vi "Group_WriteLog.vi"(0 "Group in":refnum<class "Group.lvclass">, 1 "tdms file":refnum<k34>, 7 "Loop Counter":i32, 9 "t0":timestamp, 11 "error in (no error)":errorcluster, 12 "dt per loop":dbl) -> (4 "Group out":refnum<class "Group.lvclass">, 6 "tdms file out":refnum<k34>, 15 "error out":errorcluster)   [LabVIEW 2023, in "Group.lvclass"]
doc: "A mid level VI which trickles down to call the write method on all channels within this group."
uses:
  Group.lvclass
  Group.lvclass/Group.ctl
  Channel/Channel.lvclass
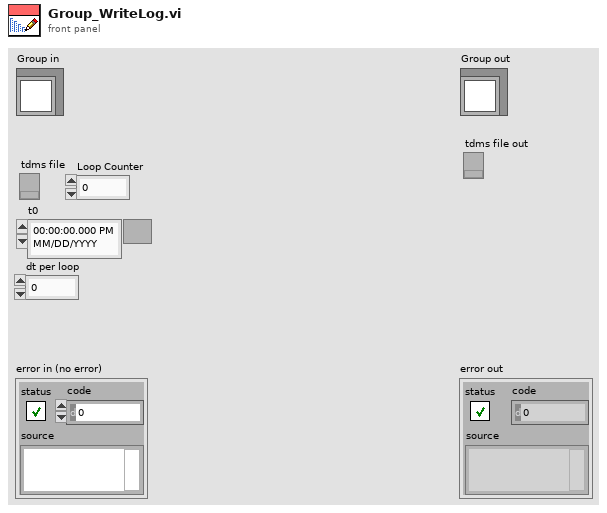
[diagram p1: front panel]
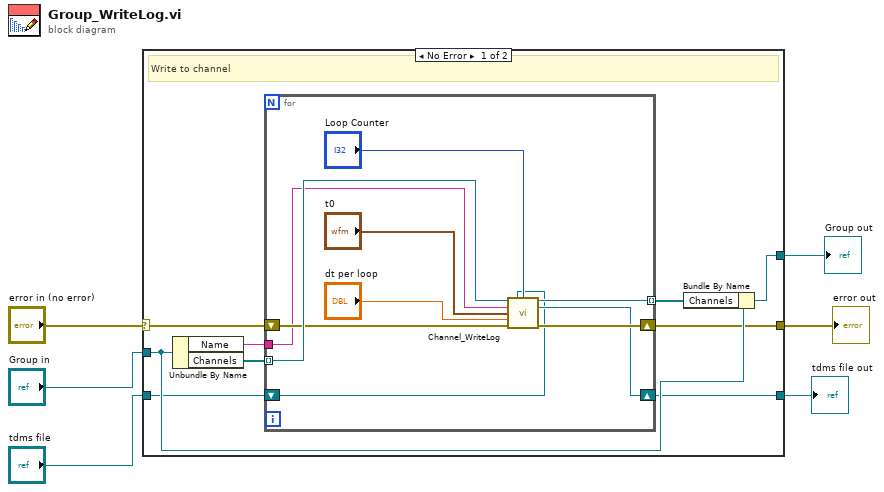
[diagram p0: block diagram]
diagram:
  n1 = case shown="No Error" "error in (no error)" {
    selector: "error in (no error)" -> [w10 w27]
    tunnel: [w11 w27] -> w5
    tunnel: [w14 w28] -> w3
    tunnel: "Group in" -> [w13 w28]
    tunnel: [w8 w26] -> w2
    tunnel: "tdms file" -> [w7 w26]
    frame No Error {
      # "Write to channel"
      n2 = Unbundle By Name(w13) -> ("Name"=w9:string, "Channels"=w15:refnum<class "Channel.lvclass">[])
      n3 = for {
        tunnel: w15 -> [w25] mode=indexing
        tunnel: [w24] -> w12 mode=indexing
        shift-right: [w23] -> w11
        shift-left: w10 -> [w22]
        tunnel: w9 -> [w18]
        shift-right: [w17] -> w8
        shift-left: w7 -> [w16]
        n4 = call-dynamic "Channel_WriteLog.vi"("Channel in"=w25, "tdms file"=w16, "Loop Counter"="Loop Counter", "Group Name"=w18, "t0"="t0", "dt per loop"="dt per loop", "error in (no error)"=w22) -> ("Channel out"=w24:refnum<class "Channel.lvclass">, "tdms file out"=w17:refnum<k34>, "error out"=w23:errorcluster)  [unwired: 6 in]
      }
      n5 = Bundle By Name(cluster=w13, "Channels"=w12) -> (w14:refnum<class "Group.lvclass">)
    }
    frame Error {
    }
  }
  "error out" <- w5
  "Group out" <- w3
  "tdms file out" <- w2
